vi "ReportHead.vi"(8 "error in (no error)":errorcluster caption="错误输入（无错误）", 11 "产品状态":string) -> (0 "error out":errorcluster caption="错误输出", 3 "report out":refnum<class "NI_report.lvclass"> caption="报表输出")   [LabVIEW 2020]
uses:
  <vilib>/Utility/NIReport.llb/NI_report.lvclass
  <vilib>/addons/_office/_exclsub.llb/font.ctl
  <vilib>/Utility/NIReport.llb/Report Type.ctl
  Global_Variable/Global.vi
  <vilib>/Utility/NIReport.llb/Append Report Text (str wrap).vi
  <vilib>/addons/_office/NI_ReportGenerationToolkit.lvlib
  <vilib>/Utility/NIReport.llb/NI_ReportGenerationCore.lvlib
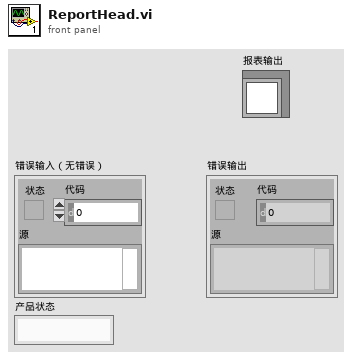
[diagram p1: front panel]
types:
  T1 = typedef "NI_ReportGenerationCore.lvlib/Report Type.ctl" = enum16{"HTML", "Word", "Excel"}
  T2 = enum16{"maximized", "minimized", "normal", "no change"}
  T3 = cluster{"操作者编号":string, "操作者姓名":string, "操作者权限":string, "联机状态":string, "产品型号":string, "产品状态":string}
  T4 = cluster{"top":dbl, "left":dbl, "right":dbl, "bottom":dbl}
  T5 = cluster{"Charset (-1)":i16, "Weight (-1)":i16, "Name":string, "Size":string}
  T6 = cluster{"Italic":enum16{"Italic Unchanged", "Italic On", "Italic Off"}, "Strike Through":enum16{"Strike Through Unchanged", "Strike Through On", "Strike Through Off"}, "Underline":enum16{"Underline Unchanged", "Underline On", "Underline Off"}, "Bold":enum16{"Bold Unchanged", "Bold On", "Bold Off"}}
  T7 = typedef "NI_ReportGenerationToolkit.lvlib/font.ctl" = cluster{"font name":string, "font size":dbl, "bold":u16, "italic":u16, "underline":u16, "strike through":u16, "font color":u32}
  T8 = cluster{"用户编号":string, "用户名":string, "用户密码(密文)":string, "用户权限":string}
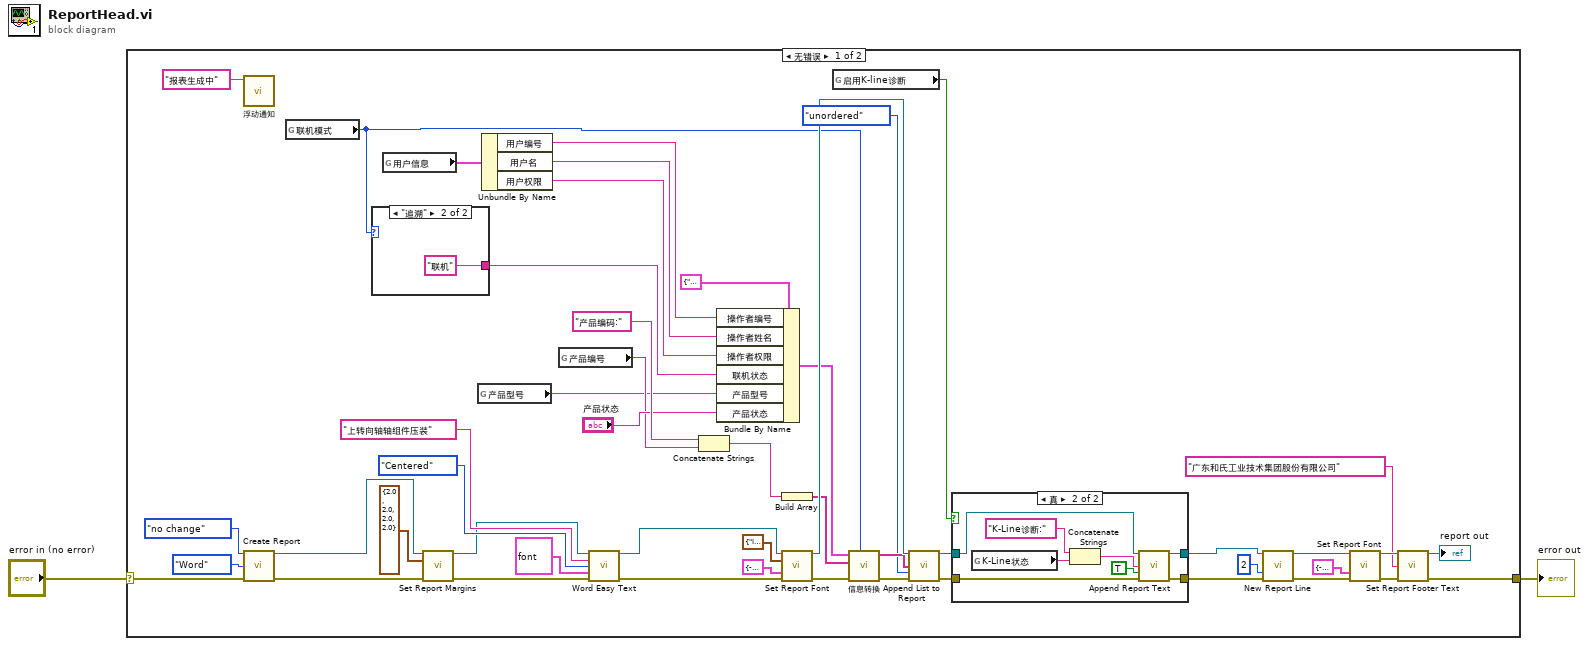
[diagram p0: block diagram]
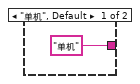
[diagram p3: hidden frame]
diagram:
  n1 = case shown="无错误" "error in (no error)" {
    selector: "error in (no error)" -> [w30 w64]
    tunnel: [w26 w64] -> w1
    frame No Error {
      n2 = call "浮动通知.vi"("通知内容"="报表生成中" ("Status")) -> ()  [unwired: 11 in]
      n3 = call <vilib>:"Create Report.vi"("window state (normal)"=T2."no change", "report type"=Report_Type."Word", "error in (no error)"=w30) -> ("report out"=w41:refnum<class "NI_report.lvclass">, "error out"=w38:errorcluster)  [unwired: 11 in]
      n4 = global read "Global.vi" "联机模式"() -> (w8:enum16{"单机", "追溯"})
      n5 = case shown="\"追溯\"" w8 {
        tunnel: ["单机" "联机"] -> w24
        frame "单机", Default {
        }
        frame "追溯" {
        }
      }
      n6 = global read "Global.vi" "用户信息"() -> (w12:T8)
      n7 = call-dynamic "Set Report Margins.vi"("report in"=w41, "margins (1.00)"=T4 {"top"=2.0, "left"=2.0, "right"=2.0, "bottom"=2.0}, "error in (no error)"=w38) -> ("report out"=w40:refnum<class "NI_report.lvclass">, "error out"=w39:errorcluster)  [unwired: 10 in, 1 out]
      n8 = global read "Global.vi" "产品型号"() -> (w15:string)
      n9 = Unbundle By Name(w12) -> ("用户编号"=w11:string, "用户名"=w10:string, "用户权限"=w9:string)
      n10 = global read "Global.vi" "产品编号"() -> (w16:string)
      n11 = call <vilib>:"Word Easy Text.vi"("report in"=w40, "text"="上转向轴轴组件压装", "alignment (left)"=enum16{"Left", "Centered", "Right", "Justify"}."Centered", "font"=T7 {"font name"="楷体", "font size"=26.0, "bold"=1, "italic"=2, "underline"=2, "strike through"=2, "font color"=16777228}, "error in (no error)"=w39) -> ("report out"=w49:refnum<class "NI_report.lvclass">, "error out"=w48:errorcluster)  [unwired: 8 in, 1 out]
      n12 = Concatenate Strings("产品编码:", w16) -> (w20:string)
      n13 = Bundle By Name(cluster=T3 {"操作者编号"="001", "操作者姓名"="Administrator", "操作者权限"="系统管理员", "联机状态"="单机", "产品型号"="SL7202", "产品状态"=""} ("测试信息"), "操作者编号"=w11, "操作者姓名"=w10, "操作者权限"=w9, "联机状态"=w24, "产品型号"=w15, "产品状态"="产品状态") -> (w22:T3)
      n14 = Build Array(w20) -> (w19:string[])
      n15 = call-dynamic "Set Report Font.vi"("report in"=w49, "text options"=T6 {"Italic"=enum."Italic Off", "Strike Through"=enum."Strike Through Unchanged", "Underline"=enum."Underline Off", "Bold"=enum."Bold Off"}, "font settings"=T5 {"Charset (-1)"=-1, "Weight (-1)"=-1, "Name"="微软雅黑 Light", "Size"="12 "}, "error in (no error)"=w48) -> ("report out"=w36:refnum<class "NI_report.lvclass">, "error out"=w29:errorcluster)  [unwired: 9 in, 1 out]
      n16 = global read "Global.vi" "启用K-line诊断"() -> (w7:bool)
      n17 = call "信息转换.vi"("联机模式"=w8, "错误输入（无错误）"=w29, "追溯码"=w19, "测试信息"=w22) -> ("错误输出"=w28:errorcluster, "信息输出"=w31:string[])  [unwired: 6 in]
      n18 = call-dynamic "Append List to Report.vi"("report in"=w36, "list elements"=w31, "list type (ordered)"=enum16{"unordered", "ordered"}."unordered", "error in (no error)"=w28) -> ("report out"=w6:refnum<class "NI_report.lvclass">, "error out"=w5:errorcluster)  [unwired: 8 in, 2 out]
      n19 = case shown="真" w7 {
        tunnel: w6 -> [w53 w58]
        tunnel: w5 -> [w52 w56]
        tunnel: [w53 w55] -> w4
        tunnel: [w52 w54] -> w3
        frame False {
        }
        frame True {
          n20 = global read "Global.vi" "K-Line状态"() -> (w60:string)
          n21 = Concatenate Strings("K-Line诊断:" ("text"), w60) -> (w59:string)
          n22 = call-poly <vilib>:"Append Report Text.vi"("report in"=w58, "text"=w59, "append on new line? (F)"=TRUE, "error in (no error)"=w56) -> ("report out"=w55:refnum<class "NI_report.lvclass">, "error out"=w54:errorcluster)  [unwired: 8 in, 2 out]
        }
      }
      n23 = call-dynamic "New Report Line.vi"("report in"=w4, "number of lines (1)"=2, "error in (no error)"=w3) -> ("report out"=w34:refnum<class "NI_report.lvclass">, "error out"=w35:errorcluster)  [unwired: 11 in]
      n24 = call-dynamic "Set Report Font.vi"("report in"=w34, "font settings"=T5 {"Charset (-1)"=-1, "Weight (-1)"=-1, "Name"="楷体", "Size"="9 "}, "error in (no error)"=w35) -> ("report out"=w45:refnum<class "NI_report.lvclass">, "error out"=w44:errorcluster)  [unwired: 10 in, 1 out]
      n25 = call-dynamic "Set Report Footer Text.vi"("report in"=w45, "center footer text"="广东和氏工业技术集团股份有限公司", "error in (no error)"=w44) -> ("report out"=→"report out":refnum<class "NI_report.lvclass">, "error out"=w26:errorcluster)  [unwired: 11 in]
    }
    frame Error {
    }
  }
  "error out" <- w1
